vi "Camera Manager Free Intptr Memory Int.vi"(8 "error in (no error)":errorcluster, 11 "imgPtr":u32) -> (0 "error out":errorcluster, 3 "imgPtr out":u32)   [LabVIEW 2017, in "PlayNitrideCameraComponet1010_4.lvlib"]
doc: "__declspec(dllexport) void CameraManager_FreeIntptrMemoryInt(unsigned int* imgPtr);"
uses:
  <userlib>/PlayNitrideCameraComponet1010_4/PlayNitrideCameraComponet1010_4.lvlib
  <userlib>/PlayNitrideCameraComponet1010_4/PlayNitrideCameraComponet.dll
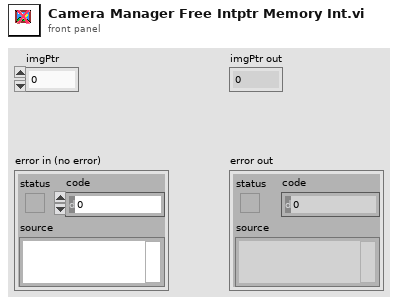
[diagram p1: front panel]
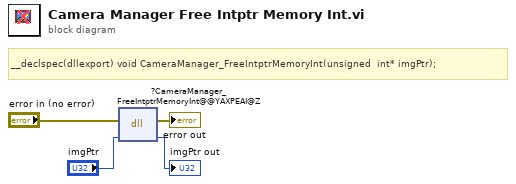
[diagram p0: block diagram]
diagram:
  # "__declspec(dllexport) void CameraManager_FreeIntptrMemoryInt(unsigned  int* imgPtr);"
  n1 = dll-call lib="C:/Program Files/National Instruments/LabVIEW 2017/user.lib/PlayNitrideCameraComponet1010_4/PlayNitrideCameraComponet.*" fn="?CameraManager_FreeIntptrMemoryInt@@YAXPEAI@Z"(error in="error in (no error)", "imgPtr"="imgPtr") -> (error out=→"error out":errorcluster, "imgPtr"=→"imgPtr out":u32)  [unwired: 3 in, 1 out]
